vi "Init.vi"(4 "Data Queue Names":string[](array[string]), 6 "Data Notifier Names":string[](array[string]), 7 "Name":string, 8 "error in (no error)":errorcluster, 10 "MSS":refnum<class "Measure and Stimulus Subsystems.lvclass">, 11 "Sample Watertemp PWM Control in":refnum<class "Sample Watertemp PWM Control.lvclass">) -> (0 "error out":errorcluster, 3 "Sample Watertemp PWM Control out":refnum<class "Sample Watertemp PWM Control.lvclass">)   [LabVIEW 2023, in "Sample Watertemp PWM Control.lvclass"]
uses:
  Sample Watertemp PWM Control.lvclass
  Sample Watertemp PWM Control.lvclass/Sample Watertemp PWM Control.ctl
  Task/Task Base/Task Base.lvclass
  Measure and Stimulus Subsystems/Measure and Stimulus Subsystems.lvclass
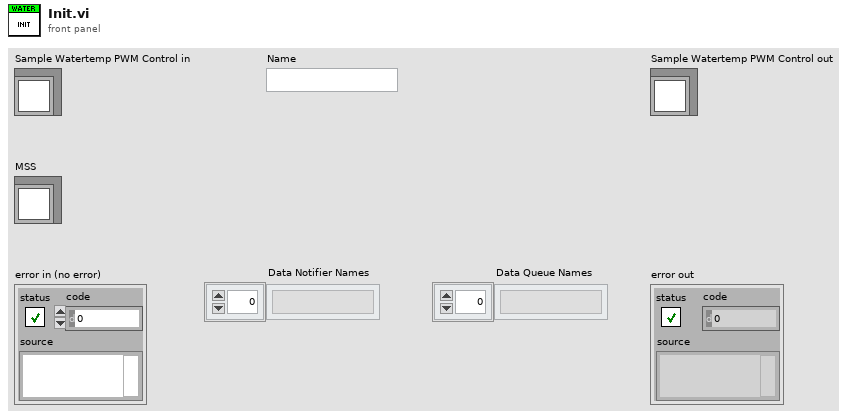
[diagram p1: front panel]
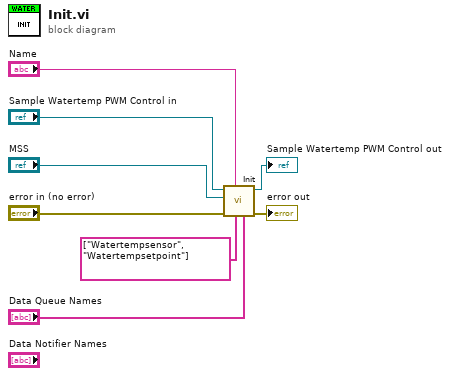
[diagram p0: block diagram]
diagram:
  n1 = call-parent "Init.vi"("Data Queue Names"="Data Queue Names", "Data Notifier Names"=string[] ["Watertempsensor", "Watertempsetpoint"], "Name"="Name", "error in (no error)"="error in (no error)", "MSS"="MSS", "Task Base in"="Sample Watertemp PWM Control in") -> ("error out"=→"error out":errorcluster, "Task Base out"=→"Sample Watertemp PWM Control out":refnum<class "Sample Watertemp PWM Control.lvclass">)  [unwired: 4 in]
